vi "Write 2D Feather Property Array.vi"(8 "error in (no error)":errorcluster, 10 "2D Feather Property Array":T1, 11 "2D Feather.lvclass in":refnum<class "2D Feather.lvclass">) -> (0 "error out":errorcluster, 3 "2D Feather.lvclass out":refnum<class "2D Feather.lvclass">)   [LabVIEW 2020, in "2D Feather.lvclass"]
uses:
  <vilib>/Math Plots/2D Math Plots/2D Feather/2D Feather/2D Feather.lvclass
  <vilib>/Math Plots/2D Math Plots/2D Feather/2D Feather/Typedef/2D Feather Property Array.ctl
  <vilib>/Math Plots/2D Math Plots/2D Feather/2D Feather/Typedef/2D Feather Property.ctl
  <vilib>/Math Plots/2D Math Plots/2D Feather/2D Feather/2D Feather.lvclass/2D Feather.ctl
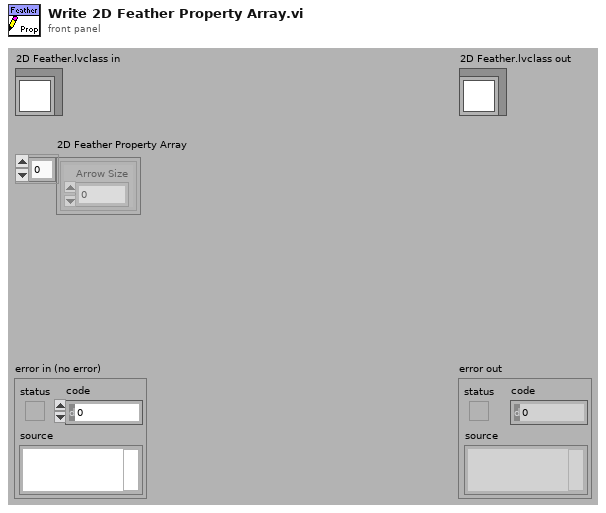
[diagram p1: front panel]
types:
  T1 = typedef "2D Feather.lvclass/2D Feather Property Array.ctl" = T2[]
  T2 = typedef "2D Feather.lvclass/2D Feather Property.ctl" = cluster{"Arrow Size":dbl}
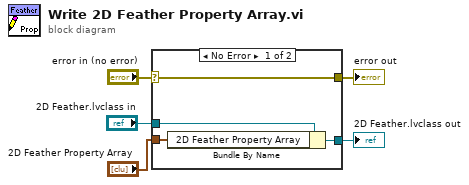
[diagram p0: block diagram]
diagram:
  n1 = case shown="No Error" "error in (no error)" {
    selector: "error in (no error)" -> [w9 w10]
    tunnel: [w9 w10] -> w4
    tunnel: [w7 w11] -> w2
    tunnel: "2D Feather.lvclass in" -> [w8 w11]
    tunnel: "2D Feather Property Array" -> [w6 _]
    frame No Error {
      n2 = Bundle By Name(cluster=w8, "2D Feather Property Array"=w6) -> (w7:refnum<class "2D Feather.lvclass">)
    }
    frame Error {
    }
  }
  "error out" <- w4
  "2D Feather.lvclass out" <- w2
